vi "Launch Views.vi"(11 "Message Enqueuer in":refnum<class "Message Enqueuer.lvclass">) -> (3 "Message Enqueuer out":refnum<class "Message Enqueuer.lvclass">)   [LabVIEW 2013]
uses:
  <vilib>/ActorFramework/Message Enqueuer/Message Enqueuer.lvclass
  <vilib>/ActorFramework/Actor/Actor.lvclass
  Views/Main View/Main View.lvclass
  Views/Project View/Project View.lvclass
  Views/Project Charm View/Project Charm View.lvclass
  Views/Create Project View/Create Project View.lvclass
  Views/Edit Project View/Edit Project View.lvclass
  Views/Sensor View/Sensor View.lvclass
  Views/Sensor Charm View/Sensor Charm View.lvclass
  Views/Create Sensor View/Create Sensor View.lvclass
  Views/Edit Sensor View/Edit Sensor View.lvclass
  Views/Test Node View/Test Node View.lvclass
  Views/Test Node Charm View/Test Node Charm View.lvclass
  Views/Create Test Node View/Create Test Node View.lvclass
  Views/Edit Test Node View/Edit Test Node View.lvclass
  <vilib>/ActorFrameworkMVC/UI Controller Messages/Launch View Actor Msg/Launch View Actor Msg.lvclass/Launch View Actor Msg.ctl
  <vilib>/ActorFramework/Message Enqueuer/Message Enqueuer.lvclass/Message Enqueuer.ctl
  <vilib>/ActorFramework/Message Enqueuer/Enqueue.vi
  <vilib>/ActorFramework/Message Priority Queue/Priority Enqueue.vi
  <vilib>/ActorFrameworkMVC/UI Controller Messages/Launch View Actor Msg/Launch View Actor Msg.lvclass
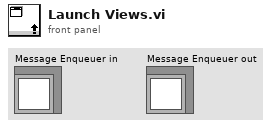
[diagram p1: front panel]
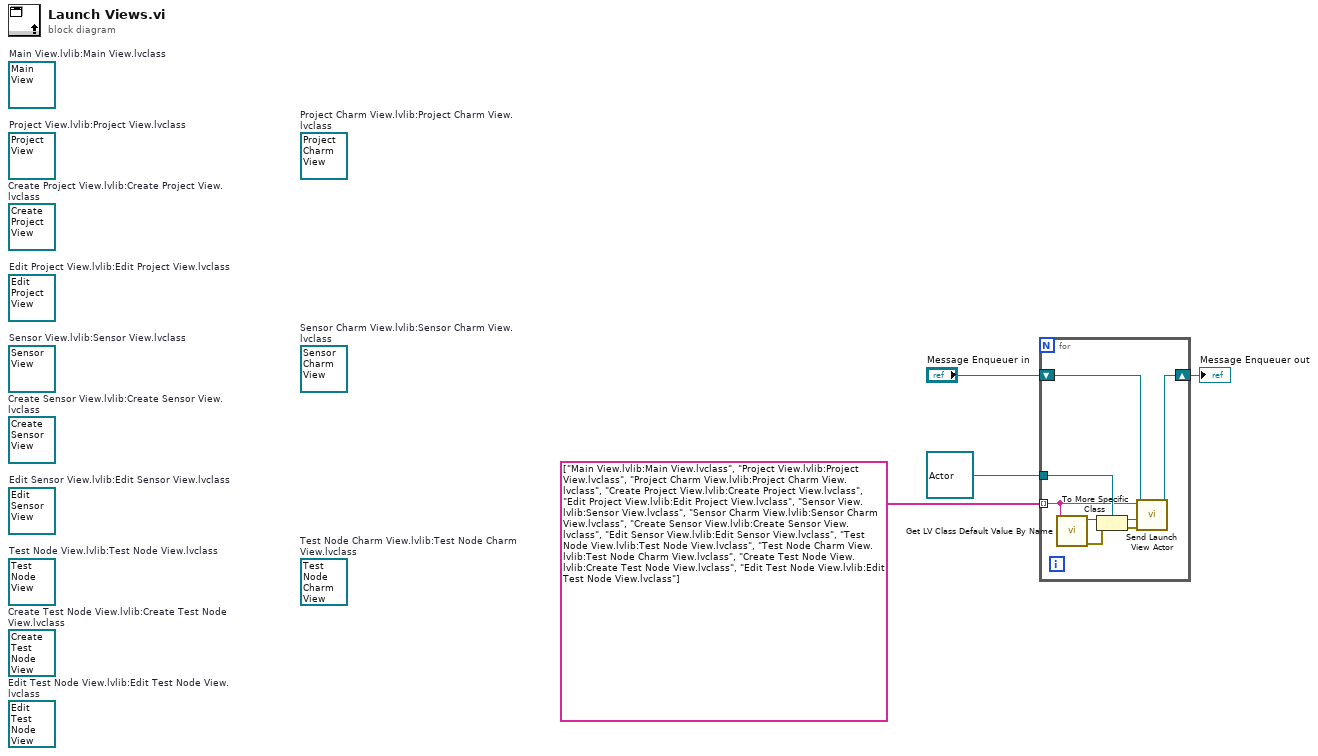
[diagram p0: block diagram]
diagram:
  (unwired) refnum<class "Edit Test Node View.lvclass"> refnum  # Edit Test Node View.lvlib:Edit Test Node View.lvclass
  (unwired) refnum<class "Create Test Node View.lvclass"> refnum  # Create Test Node View.lvlib:Create Test Node View.lvclass
  (unwired) refnum<class "Test Node Charm View.lvclass"> refnum  # Test Node Charm View.lvlib:Test Node Charm View.lvclass
  (unwired) refnum<class "Test Node View.lvclass"> refnum  # Test Node View.lvlib:Test Node View.lvclass
  (unwired) refnum<class "Edit Sensor View.lvclass"> refnum  # Edit Sensor View.lvlib:Edit Sensor View.lvclass
  (unwired) refnum<class "Create Sensor View.lvclass"> refnum  # Create Sensor View.lvlib:Create Sensor View.lvclass
  (unwired) refnum<class "Sensor Charm View.lvclass"> refnum  # Sensor Charm View.lvlib:Sensor Charm View.lvclass
  (unwired) refnum<class "Sensor View.lvclass"> refnum  # Sensor View.lvlib:Sensor View.lvclass
  (unwired) refnum<class "Edit Project View.lvclass"> refnum  # Edit Project View.lvlib:Edit Project View.lvclass
  (unwired) refnum<class "Create Project View.lvclass"> refnum  # Create Project View.lvlib:Create Project View.lvclass
  (unwired) refnum<class "Project Charm View.lvclass"> refnum  # Project Charm View.lvlib:Project Charm View.lvclass
  (unwired) refnum<class "Project View.lvclass"> refnum  # Project View.lvlib:Project View.lvclass
  (unwired) refnum<class "Main View.lvclass"> refnum  # Main View.lvlib:Main View.lvclass
  n1 = for {
    shift-right: [w7] -> w4
    shift-left: "Message Enqueuer in" -> [w9]
    tunnel: refnum<class "Actor.lvclass"> refnum ("UI Actor") -> [w12]
    tunnel: string[] ["Main View.lvlib:Main View.lvclass", "Project View.lvlib:Project View.lvclass", "Project Charm View.lvlib:Project Charm View.lvclass", "Create Project View.lvlib:Create Project View.lvclass", "Edit Project View.lvlib:Edit Project View.lvclass", "Sensor View.lvlib:Sensor View.lvclass", "Sensor Charm View.lvlib:Sensor Charm View.lvclass", "Create Sensor View.lvlib:Create Sensor View.lvclass", "Edit Sensor View.lvlib:Edit Sensor View.lvclass", "Test Node View.lvlib:Test Node View.lvclass", "Test Node Charm View.lvlib:Test Node Charm View.lvclass", "Create Test Node View.lvlib:Create Test Node View.lvclass", "Edit Test Node View.lvlib:Edit Test Node View.lvclass"] -> [w8] mode=indexing
    n2 = call <vilib>:"Get LV Class Default Value By Name.vi"("class name"=w8) -> ("error out"=w6:errorcluster, "object"=w11:refnum<class>)  [unwired: 9 in]
    n3 = To More Specific Class(target class=w12, reference=w11, error in=w6) -> (specific class reference=w10:refnum<class "Actor.lvclass">, error out=w5:errorcluster)
    n4 = call <vilib>:"Send Launch View Actor.vi"("error in (no error)"=w5, "View Actor"=w10, "View Name"=w8, "Message Enqueuer"=w9) -> ("Message Enqueuer out"=w7:refnum<class "Message Enqueuer.lvclass">)  [unwired: 6 in, 1 out]
  }
  "Message Enqueuer out" <- w4
